vi "parse rest of message.vi"(5 "timeout/kb ms (1)":i32=1, 7 "continuation timeout ms (2000)":i32=2000, 8 "error in":errorcluster, 10 "mask(1)+length(7)":u8, 11 "TCP Network Connection in":refnum<k5>) -> (0 "error out":errorcluster, 3 "unmasked data":string)   [LabVIEW 2016, in "websocket core.lvlib"]
uses:
  websocket core.lvlib
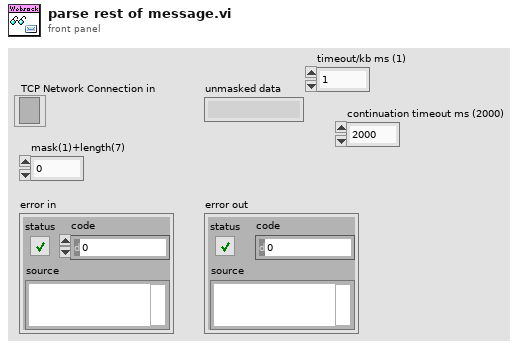
[diagram p1: front panel]
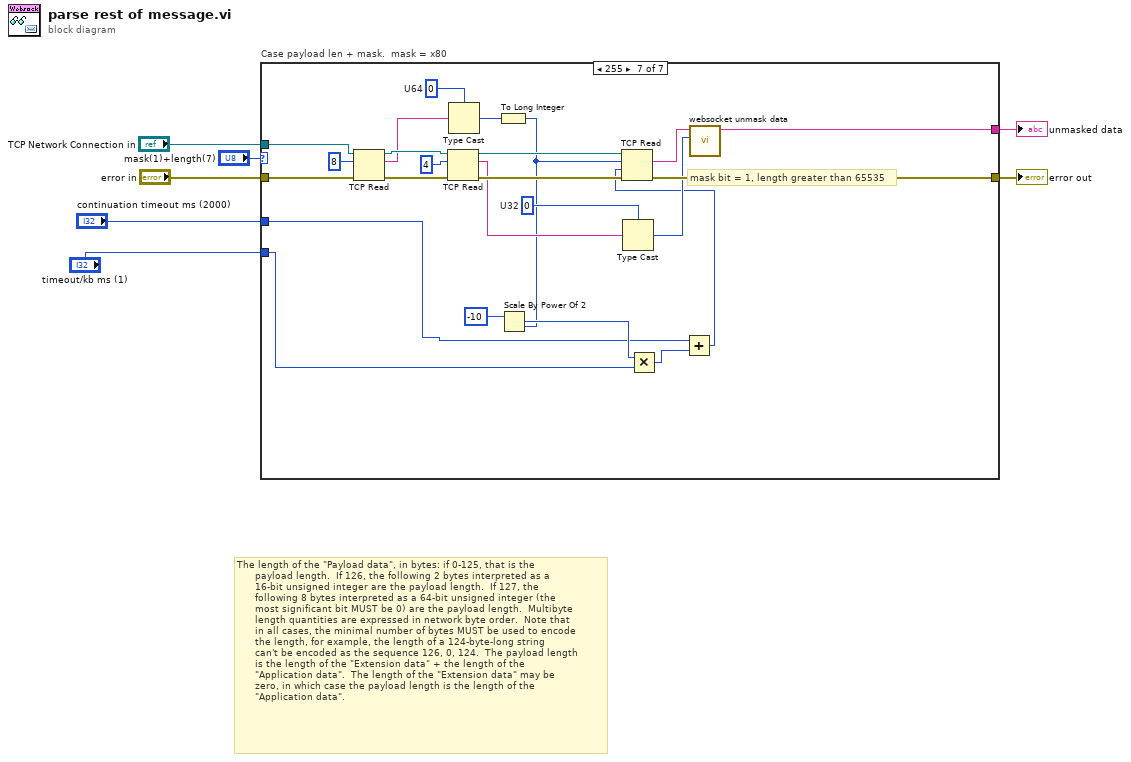
[diagram p0: block diagram]
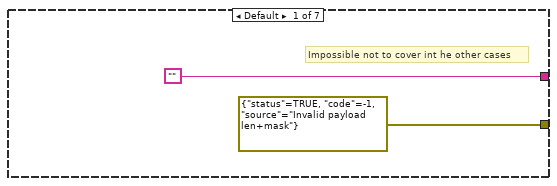
[diagram p2: hidden frame]
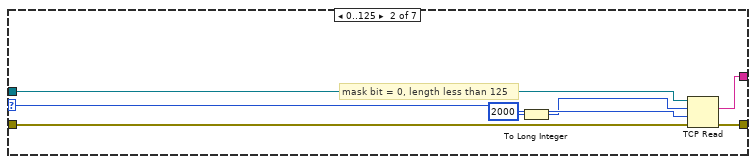
[diagram p3: hidden frame]
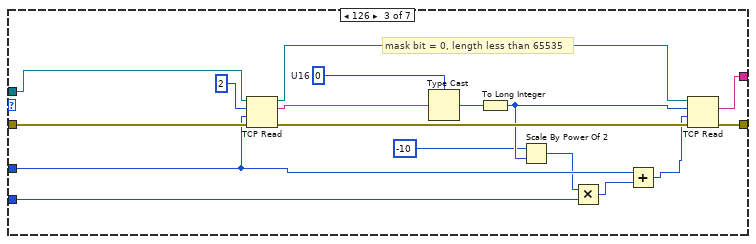
[diagram p4: hidden frame]
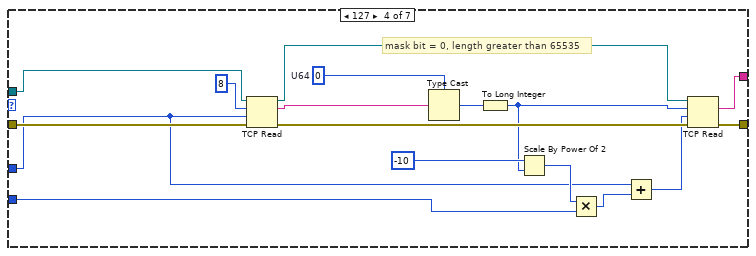
[diagram p5: hidden frame]
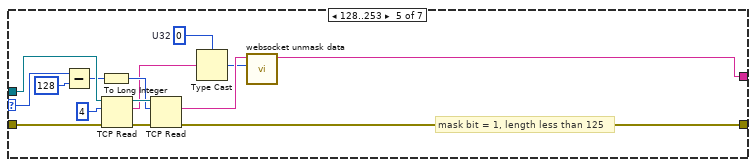
[diagram p6: hidden frame]
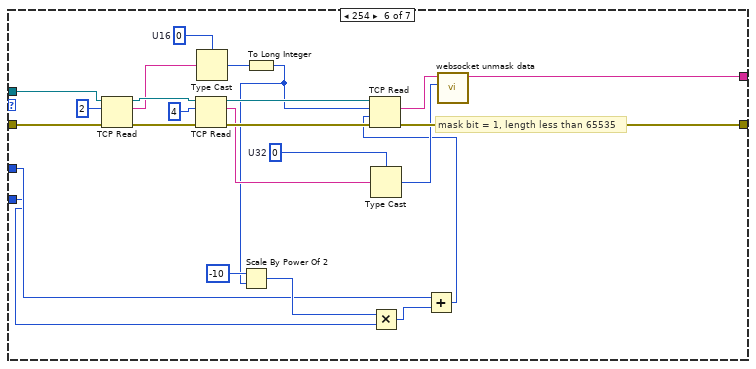
[diagram p7: hidden frame]
diagram:
  # "The length of the \"Payload data\", in bytes: if 0-125, that is the\n      payload length.  If 126, the following 2 bytes interpreted as a\n      16-bit unsigned integer are the payload length.  If 127, the\n      following 8 bytes interpreted as a 64-bit unsigned integer (the\n      most significant bit MUST be 0) are the payload length.  Multibyte\n      length quantities are expressed in network byte order.  Note that\n      in all cases, the minimal number of bytes MUST be used to encode\n      the length, for example, the length of a 124-byte-long string\n      can't be encoded as the sequence 126, 0, 124.  The payload length\n      is the length of the \"Extension data\" + the length of the\n      \"Application data\".  The length of the \"Extension data\" may be\n      zero, in which case the payload length is the length of the\n      \"Application data\"."
  n1 = case "Case payload len + mask.  mask = x80" shown="255" "mask(1)+length(7)" {
    selector: "mask(1)+length(7)" -> [_ w15 _ _ w64 _ _]
    tunnel: ["" w12 w26 w43 w53 w74 w98] -> w7
    tunnel: "TCP Network Connection in" -> [_ w16 w33 w50 w65 w89 w113]
    tunnel: [errorcluster {"status"=TRUE, "code"=-1, "source"="Invalid payload len+mask"} ("error out") w11 w25 w42 w51 w78 w103] -> w6
    tunnel: "error in" -> [_ w10 w24 w41 w55 w75 w99]
    tunnel: "continuation timeout ms (2000)" -> [_ _ w23 w34 _ w69 w92]
    tunnel: "timeout/kb ms (1)" -> [_ _ w19 w35 _ w68 w93]
    frame Default {
      # "Impossible not to cover int he other cases"
    }
    frame 0..125 {
      # "mask bit = 0, length less than 125"
      n2 = To Long Integer(number=w15) -> (32bit integer=w13:i32)
      n3 = TCP Read(connection ID=w16, bytes to read=w13, error in (no error)=w10, 9:2000 ("timeout ms (25000)")) -> (data out=w12:string, error out=w11:errorcluster)  [unwired: 1 in, 1 out]
    }
    frame 126 {
      w27 = u16 0  # U16
      # "mask bit = 0, length less than 65535"
      n4 = TCP Read(connection ID=w33, bytes to read=2, error in (no error)=w24, 9:w23) -> (connection ID out=w31:refnum<k5>, data out=w29:string, error out=w30:errorcluster)  [unwired: 1 in]
      n5 = Type Cast(type=w27, x=w29) -> (*(type *) &x=w28:u16)
      n6 = To Long Integer(number=w28) -> (32bit integer=w22:i32)
      n7 = Scale By Power Of 2(n=i16 -10, x=w22) -> (x*2^n=w20:i32)
      n8 = Multiply(x=w20, y=w19) -> (x*y=w18:i32)
      n9 = Add(x=w23, y=w18) -> (x+y=w17:i32)
      n10 = TCP Read(connection ID=w31, bytes to read=w22, error in (no error)=w30, 9:w17) -> (data out=w26:string, error out=w25:errorcluster)  [unwired: 1 in, 1 out]
    }
    frame 127 {
      w44 = u64 0  # U64
      # "mask bit = 0, length greater than 65535"
      n11 = TCP Read(connection ID=w50, bytes to read=8, error in (no error)=w41, 9:w34) -> (connection ID out=w48:refnum<k5>, data out=w46:string, error out=w47:errorcluster)  [unwired: 1 in]
      n12 = Type Cast(type=w44, x=w46) -> (*(type *) &x=w45:u64)
      n13 = To Long Integer(number=w45) -> (32bit integer=w37:i32)
      n14 = Scale By Power Of 2(n=i16 -10, x=w37) -> (x*2^n=w39:i32)
      n15 = Multiply(x=w39, y=w35) -> (x*y=w38:i32)
      n16 = Add(x=w34, y=w38) -> (x+y=w36:i32)
      n17 = TCP Read(connection ID=w48, bytes to read=w37, error in (no error)=w47, 9:w36) -> (data out=w43:string, error out=w42:errorcluster)  [unwired: 1 in, 1 out]
    }
    frame 128..253 {
      w56 = u32 0  # U32
      # "mask bit = 1, length less than 125"
      n18 = Subtract(x=w64, y=u8 128) -> (x-y=w59:u8)
      n19 = To Long Integer(number=w59) -> (32bit integer=w58:i32)
      n20 = TCP Read(connection ID=w65, bytes to read=4, error in (no error)=w55) -> (connection ID out=w61:refnum<k5>, data out=w57:string, error out=w60:errorcluster)  [unwired: 2 in]
      n21 = TCP Read(connection ID=w61, bytes to read=w58, error in (no error)=w60) -> (data out=w54:string, error out=w51:errorcluster)  [unwired: 2 in, 1 out]
      n22 = Type Cast(type=w56, x=w57) -> (*(type *) &x=w52:u32)
      n23 = call "websocket unmask data.vi"("mask key"=w52, "masked data"=w54) -> ("unmasked data"=w53:string)  [unwired: 9 in]
    }
    frame 254 {
      w76 = u32 0  # U32
      w83 = u16 0  # U16
      # "mask bit = 1, length less than 65535"
      n24 = TCP Read(connection ID=w89, bytes to read=2, error in (no error)=w75) -> (connection ID out=w87:refnum<k5>, data out=w80:string, error out=w86:errorcluster)  [unwired: 2 in]
      n25 = TCP Read(connection ID=w87, bytes to read=4, error in (no error)=w86) -> (connection ID out=w82:refnum<k5>, data out=w77:string, error out=w81:errorcluster)  [unwired: 2 in]
      n26 = Type Cast(type=w83, x=w80) -> (*(type *) &x=w84:u16)
      n27 = To Long Integer(number=w84) -> (32bit integer=w66:i32)
      n28 = Scale By Power Of 2(n=i16 -10, x=w66) -> (x*2^n=w71:i32)
      n29 = Type Cast(type=w76, x=w77) -> (*(type *) &x=w73:u32)
      n30 = Multiply(x=w71, y=w68) -> (x*y=w70:i32)
      n31 = Add(x=w69, y=w70) -> (x+y=w67:i32)
      n32 = TCP Read(connection ID=w82, bytes to read=w66, error in (no error)=w81, 9:w67) -> (data out=w79:string, error out=w78:errorcluster)  [unwired: 1 in, 1 out]
      n33 = call "websocket unmask data.vi"("mask key"=w73, "masked data"=w79) -> ("unmasked data"=w74:string)  [unwired: 9 in]
    }
    frame 255 {
      w100 = u32 0  # U32
      w107 = u64 0  # U64
      # "mask bit = 1, length greater than 65535"
      n34 = TCP Read(connection ID=w113, bytes to read=8, error in (no error)=w99) -> (connection ID out=w111:refnum<k5>, data out=w104:string, error out=w110:errorcluster)  [unwired: 2 in]
      n35 = TCP Read(connection ID=w111, bytes to read=4, error in (no error)=w110) -> (connection ID out=w106:refnum<k5>, data out=w101:string, error out=w105:errorcluster)  [unwired: 2 in]
      n36 = Type Cast(type=w107, x=w104) -> (*(type *) &x=w108:u64)
      n37 = To Long Integer(number=w108) -> (32bit integer=w91:i32)
      n38 = Scale By Power Of 2(n=i16 -10, x=w91) -> (x*2^n=w95:i32)
      n39 = Type Cast(type=w100, x=w101) -> (*(type *) &x=w97:u32)
      n40 = Multiply(x=w95, y=w93) -> (x*y=w94:i32)
      n41 = Add(x=w92, y=w94) -> (x+y=w90:i32)
      n42 = TCP Read(connection ID=w106, bytes to read=w91, error in (no error)=w105, 9:w90) -> (data out=w102:string, error out=w103:errorcluster)  [unwired: 1 in, 1 out]
      n43 = call "websocket unmask data.vi"("mask key"=w97, "masked data"=w102) -> ("unmasked data"=w98:string)  [unwired: 9 in]
    }
  }
  "unmasked data" <- w7
  "error out" <- w6
